vi "First Order Lag Filter (DBL).vi"(1 "k (1)":dbl=1.0, 2 "Raw Value in":dbl, 4 "Prev Filtered Val (Optional)":dbl=nan) -> (6 "Filtered Value out":dbl)   [LabVIEW 2018, in "RT - Analysis.lvlib"]
doc: "Performs a 1st Order Lag on a single value following the equation:\n<B>NewFilteredVal = k * RawVal + (1 - k) * OldFilteredVal</B>"
uses:
  RT - Analysis.lvlib
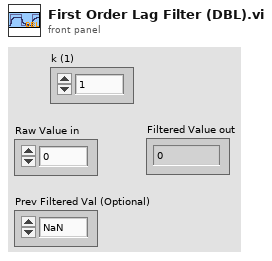
[diagram p1: front panel]
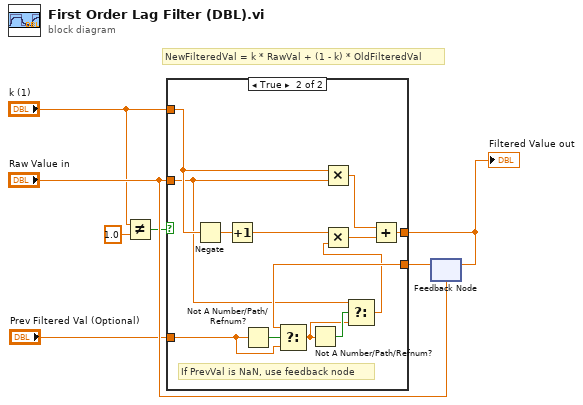
[diagram p0: block diagram]
diagram:
  # "NewFilteredVal = k * RawVal + (1 - k) * OldFilteredVal"
  n1 = Not Equal?(x="k (1)", y=1.0) -> (x != y?=w3:bool)
  n2 = feedback #1("Raw Value in") -> (w5:dbl)
  n3 = case shown="True" w3 {
    tunnel: [w8 w21] -> w7
    tunnel: "k (1)" -> [_ w18]
    tunnel: "Raw Value in" -> [w8 w11]
    tunnel: w5 -> [_ w13]
    tunnel: "Prev Filtered Val (Optional)" -> [_ w14]
    frame False {
    }
    frame True {
      # "If PrevVal is NaN, use feedback node"
      n4 = Negate(x=w18) -> (-x=w19:dbl)
      n5 = Increment(x=w19) -> (x+1=w20:dbl)
      n6 = Not A Number/Path/Refnum?(number/path/refnum=w14) -> (NaN/Path/Refnum?=w15:bool)
      n7 = Select(t=w13, s=w15, f=w14) -> (s? t:f=w10:dbl)
      n8 = Not A Number/Path/Refnum?(number/path/refnum=w10) -> (NaN/Path/Refnum?=w12:bool)
      n9 = Multiply(x=w18, y=w11) -> (x*y=w16:dbl)
      n10 = Select(t=w11, s=w12, f=w10) -> (s? t:f=w9:dbl)
      n11 = Multiply(x=w20, y=w9) -> (x*y=w17:dbl)
      n12 = Add(x=w16, y=w17) -> (x+y=w21:dbl)
    }
  }
  "Filtered Value out" <- w7
  n13 = feedback-in #1(w7) -> ()
